vi "SMO.jsonRPC.DecodeResults.vi"(7 "result type":variant, 8 "error in (no error)":errorcluster, 11 "Response in":refnum<class "Response.lvclass">) -> (0 "error out":errorcluster, 2 "id (-1: notification)":i32, 3 "result":variant)   [LabVIEW 2013, in "SMO.jsonRPC.lvclass"]
uses:
  SMO.jsonRPC.lvclass
  <vilib>/JKI/JKI JSON RPC Specification/Response/Response.lvclass
  <vilib>/JKI/JKI JSON RPC Specification/Response/Response.lvclass/Response.ctl
  <vilib>/JKI/JKI JSON RPC Specification/Error/Error.lvclass/Error.ctl
  <vilib>/JKI/JKI JSON RPC Specification/Error/Error.lvclass
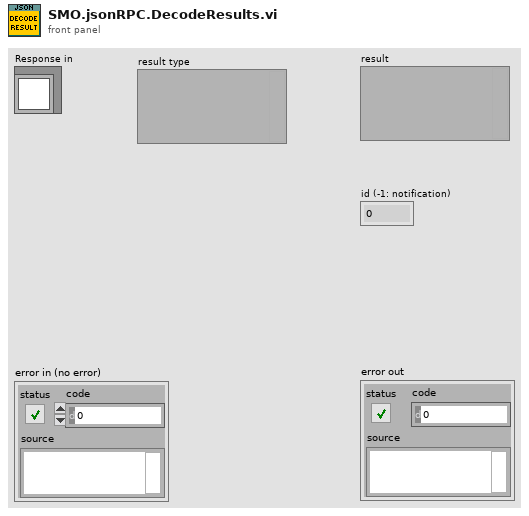
[diagram p1: front panel]
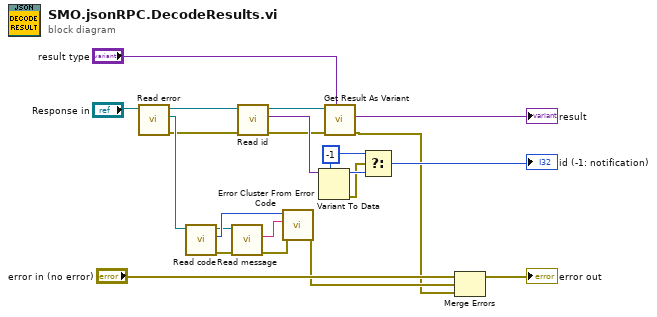
[diagram p0: block diagram]
diagram:
  w19 = -1 ("id (-1: notification)")
  n1 = call <vilib>:"Read error.vi"("Response in"="Response in") -> ("error out"=w9:errorcluster, "Error"=w11:refnum<class "Error.lvclass">, "Response out"=w8:refnum<class "Response.lvclass">)  [unwired: 8 in]
  n2 = call <vilib>:"Read code.vi"("Error in"=w11) -> ("error out"=w12:errorcluster, "code"=w14:i16, "Error out"=w13:refnum<class "Error.lvclass">)  [unwired: 8 in]
  n3 = call <vilib>:"Read message.vi"("error in (no error)"=w12, "Error in"=w13) -> ("error out"=w16:errorcluster, "message"=w15:string)  [unwired: 7 in, 1 out]
  n4 = call <vilib>:"Read id.vi"("error in (no error)"=w9, "Response in"=w8) -> ("error out"=w5:errorcluster, "id"=w6:variant, "Response out"=w4:refnum<class "Response.lvclass">)  [unwired: 7 in]
  n5 = call <vilib>:"Error Cluster From Error Code.vi"("error in (no error)"=w16, "error message (\"\")"=w15, "error code (0)"=w14) -> ("error out"=w17:errorcluster)  [unwired: 6 in]
  n6 = Variant To Data(type=w19, Variant=w6) -> (data=w20:i32, error out=w18:errorcluster)  [unwired: 1 in]
  n7 = call <vilib>:"Get Result As Variant.vi"("type"="result type", "error in (no error)"=w5, "Response in"=w4) -> ("error out"=w2:errorcluster, "result"=→"result":variant)  [unwired: 6 in, 1 out]
  n8 = Select(t=w19, s=w18, f=w20) -> (s? t:f=→"id (-1: notification)":i32)
  n9 = Merge Errors("error in (no error)", w17, w2) -> (→"error out":errorcluster)
